vi "MM6.PG_getConfigKnorz.vi"(0 "i ref in":refnum<vi>, 5 "error in (no error)":errorcluster) -> (14 "i ref out":refnum<vi>, 16 "PGData":T1, 19 "error out":errorcluster)   [LabVIEW 2014, in "MM6.lvlib"]
doc: "This is real \"Knorz\". Try to get the trigger stuff from the database (via the BaseProcess attribute), analyze the attribute data of this class to get the \"memory\" configuration.\n\nFirst, a better solution would be to obtain the trigger conditions not via the database but via user input. \nSecond, the number of the actual configuration (for a \"switch measurement\") needs to be implemented."
uses:
  MM6.lvlib
  CS_DigitalIO/PPG_ABC/PPG_ABC.PG_dataType.ctl
  CS_Core/BaseProcess/BaseProcess.lvlib
  LEBITLib/LEBITLib.lvlib
  CS_DigitalIO/PPG_ABC/PPG_ABC.lvlib
panel:
  in  "PGDataType":T1
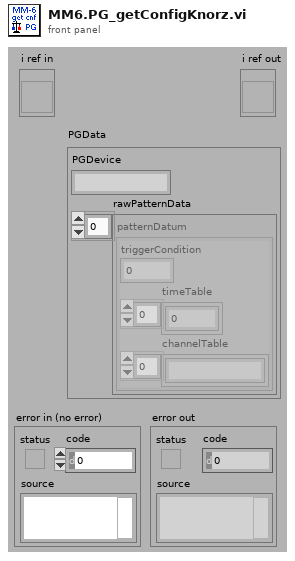
[diagram p1: front panel]
types:
  T1 = typedef "PPG_ABC.lvlib/PPG_ABC.PG_dataType.ctl" = cluster{"PGDevice":string, "rawPatternData":cluster{"triggerCondition":i32, "timeTable":dbl[], "channelTable":string[]}[]}
  T2 = typedef "BaseProcess.lvlib/BaseProcess.i attribute.ctl" = cluster{"EventStatus":string, "EventError":i32, "PresetEvtWatchD":i32, "PresetPdcWatchD":i32, "EventTimeout":i32, "PeriodicInterval":i32, "Interface":string[], "Address":string[], "Special":string[], "PeriodicError":i32, "PeriodicStatus":string, "SuperProc":string, "Descriptors":T3[], "CaseRef":refnum<vi>, "PdcRef":refnum<vi>, "Thread Ref":refnum<vi>, "eventErrorID":i32, "eventStatusID":i32, "periodicErrorID":i32, "periodicStatusID":i32, "pdcCtrID":i32}
  T3 = typedef "BaseProcess.lvlib/BaseProcess.descriptor definition.ctl" = cluster{"selector":string, "descriptor":T4}
  T4 = typedef "BaseProcess.lvlib/BaseProcess.descriptor string definition.ctl" = string
  T5 = typedef "MM6.lvlib/MM6.i attribute.ctl" = cluster{"ConfigData":T6, "UsedObjs":string[], "ActScanStep":i32[], "AbortRequest":bool, "StopRequest":bool, "# cycles":i32, "Connected":bool, "MMStatus":T21, "# data":i32, "DIMServices":cluster{"MM6StatusString":string, "MM6StatusID":i32, "discArchiver":string, "discArchiverID":i32, "eventBuilder":string, "eventBuilderID":i32, "GUIIDString":string, "GUIIDStringID":i32}, "dataFile":string, "ExtraDataSets":T22, "PGRunning":T23}
  T6 = typedef "LEBITDefs.lvlib/LEBITDefs.ConfigData.ctl" = cluster{"GenConfig":T7, "Configs":T9[]}
  T7 = typedef "LEBITDefs.lvlib/LEBITDefs.GenConfig.ctl" = cluster{"Mode":i32, "Logs":T8[]}
  T8 = typedef "LEBITDefs.lvlib/LEBITDefs.Log.ctl" = cluster{"Name":string, "FctName":string, "Special":string}
  T9 = typedef "LEBITDefs.lvlib/LEBITDefs.OneConfig.ctl" = cluster{"MCA":T10, "Timing":T11, "Scans":T14[], "FreqDevs":T15[], "CleanDev":T16, "NrCycles":i32, "Specials":T18[], "Delays":T19[], "DAC":T20}
  T10 = typedef "LEBITDefs.lvlib/LEBITDefs.MCA.ctl" = cluster{"Name":string, "Address":string, "NrChannels":i32, "Gate":i32, "NrPipse":i32}
  T11 = typedef "LEBITDefs.lvlib/LEBITDefs.Timing.ctl" = cluster{"TimeTables":cluster{"TimeTable":T12}[], "Memories":T13[], "ScanX":string, "ScanY":string}
  T12 = typedef "LEBITDefs.lvlib/LEBITDefs.Timetable.ctl" = dbl[]
  T13 = typedef "LEBITDefs.lvlib/LEBITDefs.Memory.ctl" = cluster{"Device":string, "ExtTrig":bool, "TT2Use":i32, "PatternTable":string[]}
  T14 = typedef "LEBITDefs.lvlib/LEBITDefs.ScanDev.ctl" = cluster{"Name":string, "FctName":string, "Values":dbl[], "NrScanVals":i32, "Special":string}
  T15 = typedef "LEBITDefs.lvlib/LEBITDefs.FreqDev.ctl" = cluster{"Name":string, "Amp":dbl, "CenterFreq":dbl, "Time":dbl}
  T16 = typedef "LEBITDefs.lvlib/LEBITDefs.CleanDev.ctl" = cluster{"Name":string, "CleanData":T17[]}
  T17 = typedef "LEBITDefs.lvlib/LEBITDefs.CleanDataType.ctl" = cluster{"Amp":dbl, "Center":dbl, "Plus":dbl, "Minus":dbl, "Time":dbl}
  T18 = typedef "LEBITDefs.lvlib/LEBITDefs.Special.ctl" = cluster{"Name":string, "FctName":string, "VerySpecial":string, "Data":dbl}
  T19 = typedef "LEBITDefs.lvlib/LEBITDefs.Delay.ctl" = cluster{"Name":string, "Delay":dbl}
  T20 = typedef "LEBITDefs.lvlib/LEBITDefs.DAC.ctl" = cluster{"Name":string, "Step1":i32, "Step2":i32}
  T21 = typedef "MM6.lvlib/MM6.status.ctl" = enum16{"loaded", "load_error", "config", "config_error", "init", "init_error", "data_reset", "data_reset_error", "running", "start_error", "run_error", "abort_requested", "aborted", "stop_requested", "stopped", "stop_error", "Connected", "NOTConnected"}
  T22 = typedef "LEBITDefs.lvlib/LEBITDefs.ExtraData.ctl" = cluster{"Ions":cluster{"ExcitIonMass":string, "ExcitIonCharge":i32, "CleanIons":cluster{"CleanIonMass":string, "CleanIonCharge":i32}[]}, "TimingDescription":cluster{"TimeTableDescription":cluster{"Times":string[]}[], "PatternTableDescription":cluster{"Pattern":string[]}[]}, "ScanUnits":string[]}[]
  T23 = typedef "PPG_ABC.lvlib/PPG_ABC.PG_Running.ctl" = i32
  T24 = cluster{"triggerCondition":i32, "timeTable":dbl[], "channelTable":string[]}[]
  T25 = cluster{"triggerCondition":i32, "timeTable":dbl[], "channelTable":string[]}
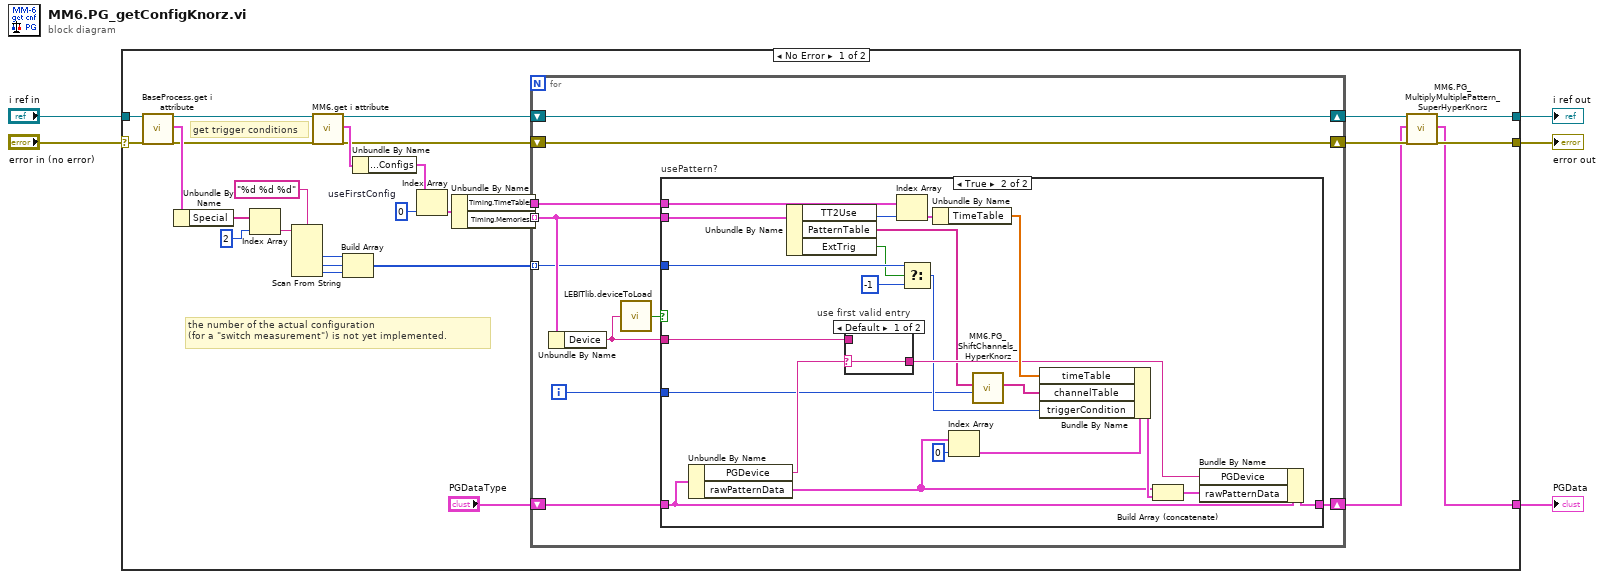
[diagram p0: block diagram]
diagram:
  n1 = case shown="No Error" "error in (no error)" {
    selector: "error in (no error)" -> [w29 w69]
    tunnel: "i ref in" -> [w33 w70]
    tunnel: [w10 w70] -> w4
    tunnel: [w8 w69] -> w3
    tunnel: [w6 _] -> w1
    frame No Error {
      w22 = 0  # useFirstConfig
      # "the number of the actual configuration \n(for a \"switch measurement\") is not yet implemented."
      # "get trigger conditions"
      n2 = call "BaseProcess.get i attribute.vi"("i ref in"=w33, "error in (no error)"=w29) -> ("i ref out"=w24:refnum<vi>, "i attribute"=w32:T2, "error out"=w25:errorcluster)  [unwired: 15 in]
      n3 = Unbundle By Name(w32) -> ("Special"=w31:string[])
      n4 = Index Array(array=w31, index=2) -> (element=w28:string)
      n5 = Scan From String(format string="%d %d %d", input string=w28) -> (output 1=w15:i32, output 2=w14:i32, output 3=w13:i32)  [unwired: 5 in, 3 out]
      n6 = call "MM6.get i attribute.vi"("i ref in"=w24, "error in (no error)"=w25) -> ("i ref out"=w20:refnum<vi>, "i attribute"=w26:T5, "error out"=w19:errorcluster)  [unwired: 15 in]
      n7 = Build Array(w15, w14, w13) -> (w12:i32[])
      n8 = Unbundle By Name(w26) -> ("ConfigData.Configs"=w23:T9[])
      n9 = Index Array(array=w23, index=w22) -> (element=w21:T9)
      n10 = Unbundle By Name(w21) -> ("Timing.TimeTables"=w17:cluster{"TimeTable":T12}[], "Timing.Memories"=w16:T13[])
      n11 = for {
        shift-right: [w36] -> w11
        shift-left: w20 -> [w36]
        shift-right: [w35] -> w9
        shift-left: w19 -> [w35]
        shift-right: [w37] -> w7
        shift-left: "PGDataType" -> [w38]
        tunnel: w17 -> [w41]
        tunnel: w16 -> [w40] mode=indexing
        tunnel: w12 -> [w39] mode=indexing
        i -> [w34]
        n12 = Unbundle By Name(w40) -> ("Device"=w42:string)
        n13 = call "LEBITlib.deviceToLoad.vi"("DeviceName"=w42) -> ("DeviceIsToLoad"=w43:bool)
        n14 = case "usePattern?" shown="True" w43 {
          tunnel: w40 -> [_ w63]
          tunnel: w42 -> [_ w64]
          tunnel: w41 -> [_ w62]
          tunnel: w39 -> [_ w51]
          tunnel: w38 -> [w44 w54]
          tunnel: [w44 w52] -> w37
          tunnel: w34 -> [_ w45]
          frame False {
          }
          frame True {
            n15 = Unbundle By Name(w54) -> ("PGDevice"=w56:string, "rawPatternData"=w57:T24)
            n16 = Unbundle By Name(w63) -> ("TT2Use"=w61:i32, "PatternTable"=w47:string[], "ExtTrig"=w50:bool)
            n17 = case "use first valid entry" shown="Default" w56 {
              selector: w56 -> [w67 _]
              tunnel: w64 -> [_ w68]
              tunnel: [w67 w68] -> w53
              frame Default {
              }
              frame "" {
              }
            }
            n18 = Index Array(array=w62, index=w61) -> (element=w60:cluster{"TimeTable":T12})
            n19 = Select(t=w51, s=w50, f=-1) -> (s? t:f=w48:i32)
            n20 = Unbundle By Name(w60) -> ("TimeTable"=w59:T12)
            n21 = Index Array(array=w57, index=0) -> (element=w65:T25)
            n22 = call "MM6.PG_ShiftChannels_HyperKnorz.vi"("patternNumber"=w45, "PatternTable"=w47) -> ("PatternTableShifted"=w46:string[])  [unwired: 9 in]
            n23 = Bundle By Name(cluster=w65, "timeTable"=w59, "channelTable"=w46, "triggerCondition"=w48) -> (w58:T25)
            n24 = Build Array (concatenate)(w57, w58) -> (w55:T24)
            n25 = Bundle By Name(cluster=w54, "PGDevice"=w53, "rawPatternData"=w55) -> (w52:T1)
          }
        }
      }
      n26 = call "MM6.PG_MultiplyMultiplePattern_SuperHyperKnorz.vi"("i ref in"=w11, "PGDataType"=w7, "error in (no error)"=w9) -> ("i ref out"=w10:refnum<vi>, "PGData"=w6:T1, "error out"=w8:errorcluster)  [unwired: 14 in]
    }
    frame Error {
    }
  }
  "error out" <- w3
  "i ref out" <- w4
  "PGData" <- w1
